vi "SS_CreateLocalFileSub.vi"(7 "Main Cluster IN":T1, 8 "Error IN":errorcluster, 9 "Number of Channels":i32, 11 "Data Array IN":string[][](array[string])) -> (0 "Error OUT":errorcluster, 3 "Data Array OUT":string[][](array[string]))   [LabVIEW 2016]
uses:
  Control/Control_Main.ctl
  Control/Control_ModuleArray.ctl
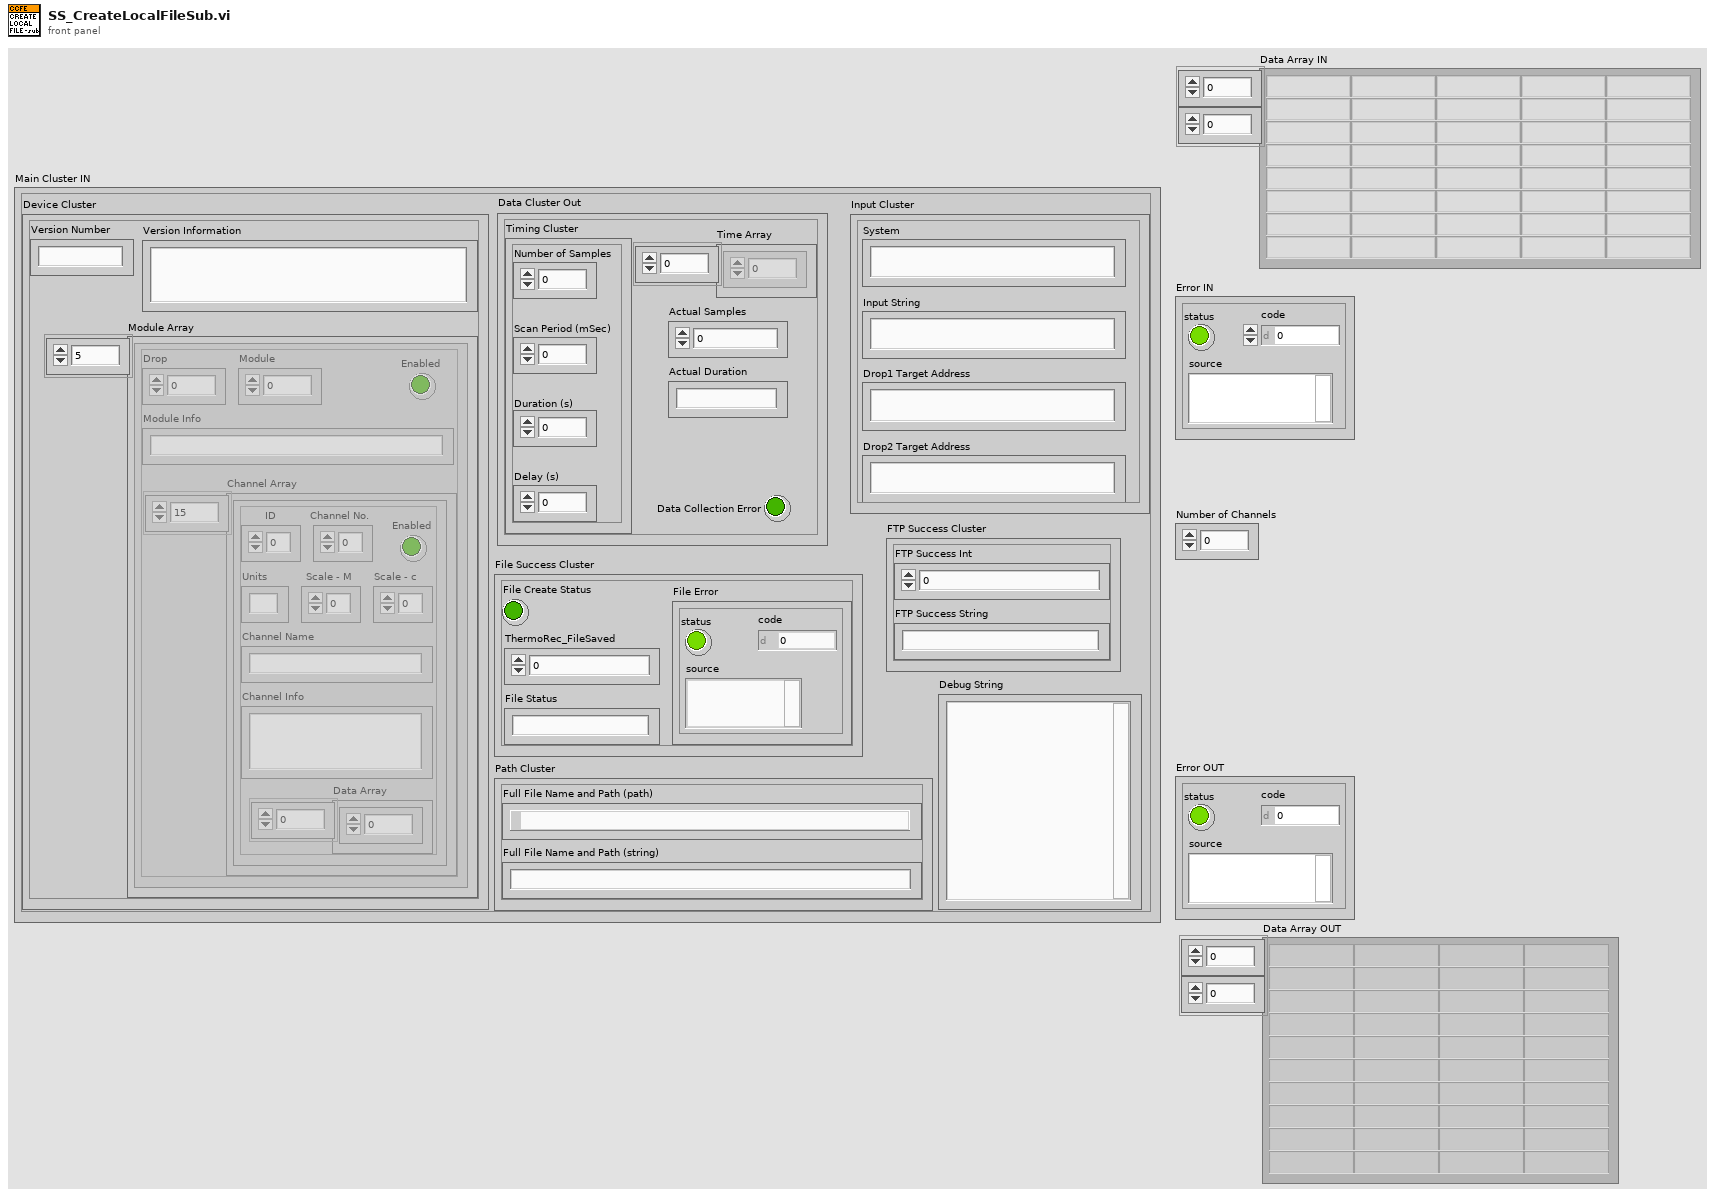
[diagram p1: front panel]
types:
  T1 = typedef "Control_Main.ctl" = cluster{"Device Cluster":cluster{"Module Array":T2, "Version Number":string, "Version Information":string}, "Input Cluster":cluster{"Input String":string, "Drop1 Target Address":string, "Drop2 Target Address":string, "System":string}, "Data Cluster Out":cluster{"Timing Cluster":cluster{"Number of Samples":i32, "Scan Period (mSec)":u32, "Duration (s)":dbl, "Delay (s)":dbl}, "Time Array":dbl[], "Actual Samples":i32, "Actual Duration":string, "Data Collection Error":bool}, "Path Cluster":cluster{"Full File Name and Path (path)":path, "Full File Name and Path (string)":string}, "File Success Cluster":cluster{"ThermoRec_FileSaved":i32, "File Create Status":bool, "File Error":errorcluster, "File Status":string}, "FTP Success Cluster":cluster{"FTP Success Int":i32, "FTP Success String":string}, "Debug String":string}
  T2 = typedef "Control_ModuleArray.ctl" = cluster{"Drop":i32, "Module":i32, "Module Info":string, "Enabled":bool, "Channel Array":cluster{"ID":i32, "Channel No.":i32, "Enabled":bool, "Channel Name":string, "Channel Info":string, "Units":string, "Scale - M":dbl, "Scale - c":dbl, "Data Array":dbl[]}[]}[]
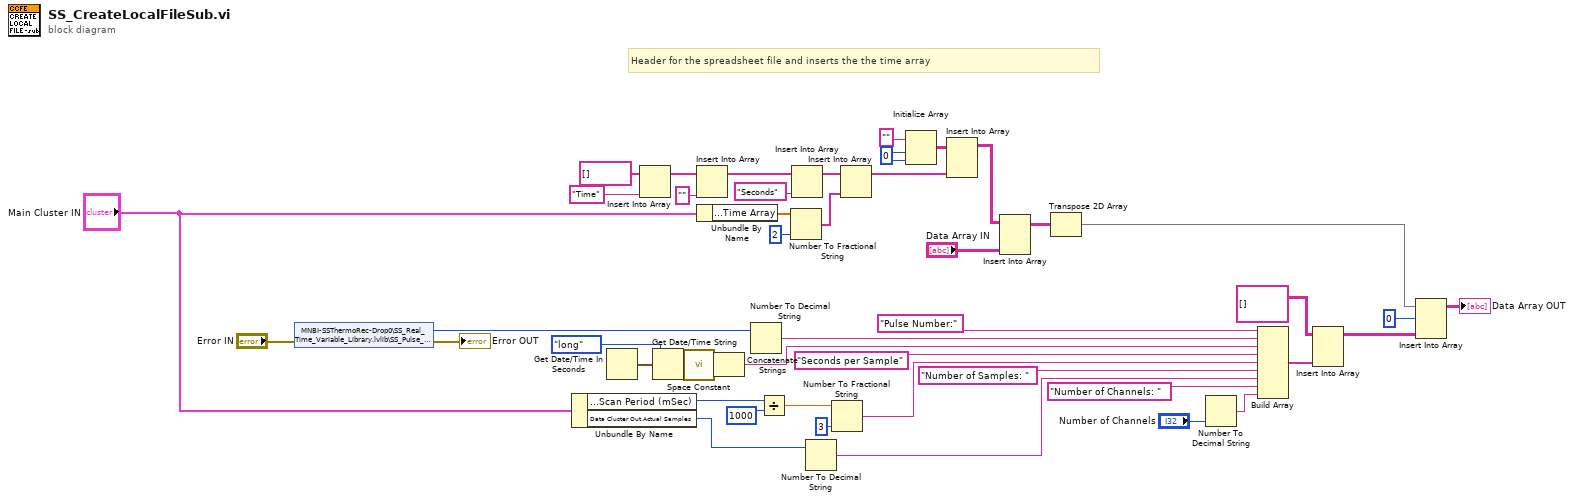
[diagram p0: block diagram]
diagram:
  w9 = 0
  # "Header for the spreadsheet file and inserts the the time array"
  n1 = shared-variable "MNBI-SSThermoRec-Drop0\\SS_Real_Time_Variable_Library.lvlib\\SS_Pulse_Number"(error in="Error IN") -> (w43:i32, error out=→"Error OUT":errorcluster)
  n2 = Unbundle By Name("Main Cluster IN") -> ("Data Cluster Out.Timing Cluster.Scan Period (mSec)"=w45:u32, "Data Cluster Out.Actual Samples"=w46:i32)
  n3 = Get Date/Time In Seconds() -> (seconds since 1Jan1904=w40:timestamp)
  n4 = Insert Into Array(array=string[] [], new element="Time" ("new element/subarray")) -> (w14:string[])  [unwired: 1 in]
  n5 = Get Date/Time String(date format (0)=enum16{"short", "long", "abbreviated"}."long", seconds (now)=w40) -> (date string=w39:string, time string=w38:string)  [unwired: 1 in]
  n6 = call <vilib>:"Space Constant.vi"() -> ("String"=w31:string)
  n7 = Insert Into Array(array=w14, new element="" ("new element/subarray")) -> (w17:string[])  [unwired: 1 in]
  n8 = Unbundle By Name("Main Cluster IN") -> ("Data Cluster Out.Time Array"=w7:dbl[])
  n9 = Concatenate Strings(w39, w31, w38) -> (w30:string)
  n10 = Number To Decimal String(number=w43) -> (decimal integer string=w32:string)  [unwired: 1 in]
  n11 = Divide(x=w45, y=u32 1000) -> (x/y=w27:dbl)
  n12 = Number To Fractional String(number=w7, precision (6)=i16 2) -> (F-format string=w19:string[])  [unwired: 2 in]
  n13 = Insert Into Array(array=w17, new element="Seconds" ("new element/subarray")) -> (w18:string[])  [unwired: 1 in]
  n14 = Number To Decimal String(number=w46) -> (decimal integer string=w24:string)  [unwired: 1 in]
  n15 = Number To Fractional String(number=w27, precision (6)=i16 3) -> (F-format string=w26:string)  [unwired: 2 in]
  n16 = Insert Into Array(array=w18, new element=w19) -> (w20:string[])  [unwired: 1 in]
  n17 = Initialize Array("", w9, w9) -> (w10:string[][])
  n18 = Insert Into Array(array=w10, new element=w20) -> (w11:string[][])  [unwired: 2 in]
  n19 = Insert Into Array(array=w11, new element="Data Array IN") -> (w42:string[][])  [unwired: 2 in]
  n20 = Transpose 2D Array(2D array=w42) -> (transposed array=w1:string[][])
  n21 = Number To Decimal String(number="Number of Channels") -> (decimal integer string=w22:string)  [unwired: 1 in]
  n22 = Build Array("Pulse Number:", w32, w30, "Seconds per Sample", w26, "Number of Samples: ", w24, "Number of Channels: ", w22) -> (w33:string[])
  n23 = Insert Into Array(array=string[][] [] ("output array 2"), new element=w33) -> (w3:string[][])  [unwired: 2 in]
  n24 = Insert Into Array(array=w1, index (row)=0, new element=w3) -> (→"Data Array OUT":string[][])  [unwired: 1 in]
